vi "Try Parse.vi"(0 "Scalar Path in":refnum<class "Scalar Path.lvclass">, 5 "Config Row":string[](array[string]), 11 "error in (no error)":errorcluster) -> (4 "Scalar Path out":refnum<class "Scalar Path.lvclass">, 6 "Is of type?":bool, 15 "error out":errorcluster)   [LabVIEW 2023, in "RFFixtureCharact.Public.lvlib" / "Scalar Path.lvclass"]
uses:
  Scalar Path.lvclass
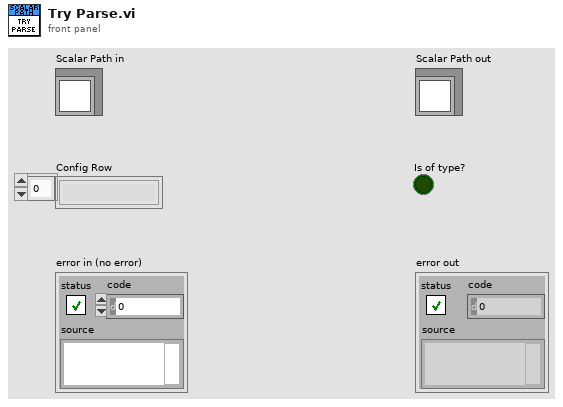
[diagram p1: front panel]
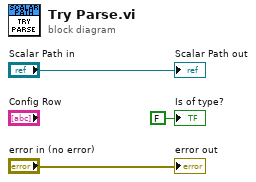
[diagram p0: block diagram]
diagram:
  "error out" <- "error in (no error)"
  "Scalar Path out" <- "Scalar Path in"
  "Is of type?" <- FALSE ("Is of type?")
